vi "getPrinterConfig.vi"(8 "Error In":errorcluster, 11 "Config File Path":path) -> (0 "Error Out":errorcluster, 3 "comPort":string)   [LabVIEW 2018]
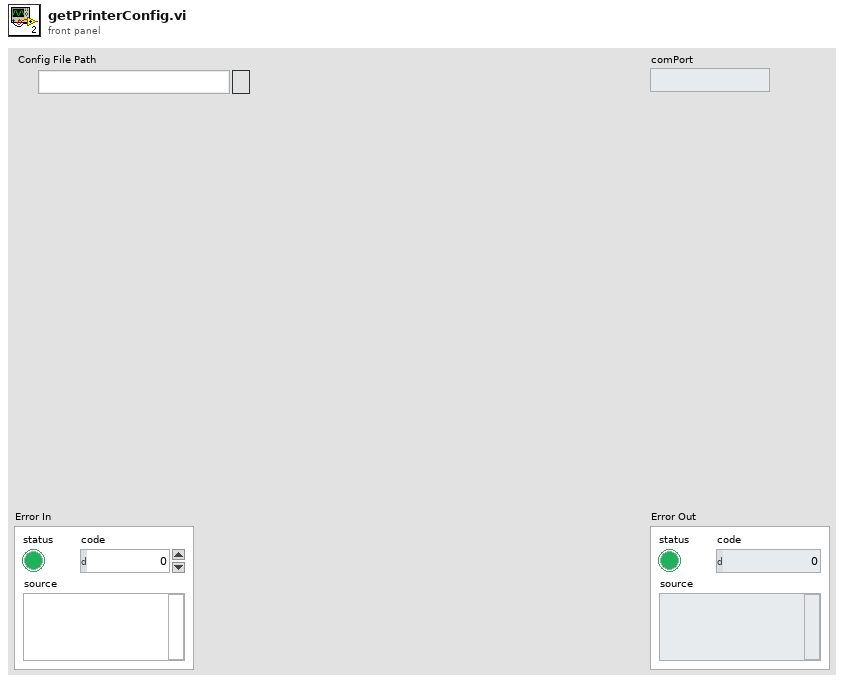
[diagram p1: front panel]
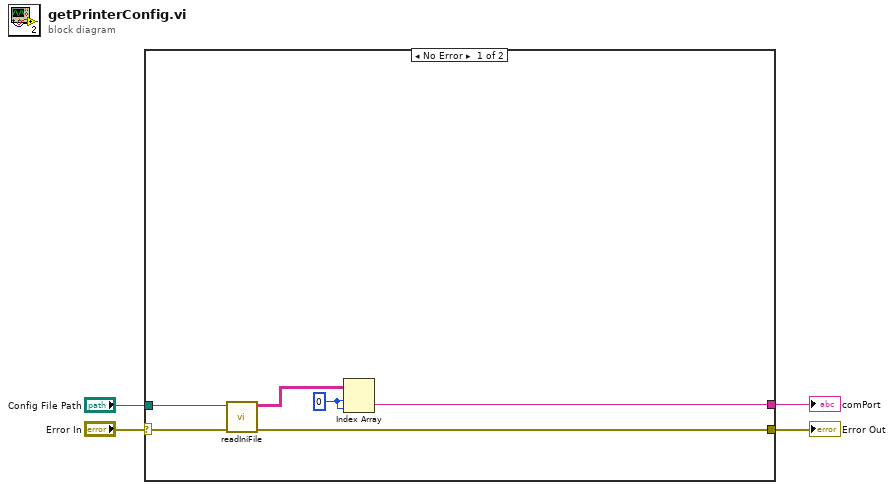
[diagram p0: block diagram]
diagram:
  n1 = case shown="No Error" "Error In" {
    selector: "Error In" -> [w8 w11]
    tunnel: [w7 w11] -> w3
    tunnel: "Config File Path" -> [w6 _]
    tunnel: [w9 _] -> w1
    frame No Error {
      w10 = 0 ("index (row)")
      n2 = call "readIniFile.vi"("Error In"=w8, "File Path Control"=w6) -> ("Error Out"=w7:errorcluster, "Value"=w5:string[][])  [unwired: 8 in]
      n3 = Index Array(array=w5, index (row)=w10, index (col)=w10) -> (element=w9:string)
    }
    frame Error {
    }
  }
  "Error Out" <- w3
  "comPort" <- w1
